vi "Database - Read.vi"(8 "error in (no error)":errorcluster, 11 "View Model":T1) -> (0 "error out":errorcluster, 3 "View Model":T1)   [LabVIEW 2017]
doc: "Reads the Configuration Database and store the information in an appropriate data structure.\n[Covers: SD3]"
uses:
  View Model/Controls/View Model.ctl
  View Model/Controls/Shared Model.ctl
  Error Handler/Controls/Error Model.ctl
  Error Handler/Controls/Error Message.ctl
  Error Handler/Controls/Error Level.ctl
  Controls/Database Model.ctl
  Controls/Database Message.ctl
  Controls/Database Command.ctl
  Controls/Database Overhead.ctl
  Controls/Database Status.ctl
  Controls/Database Record.ctl
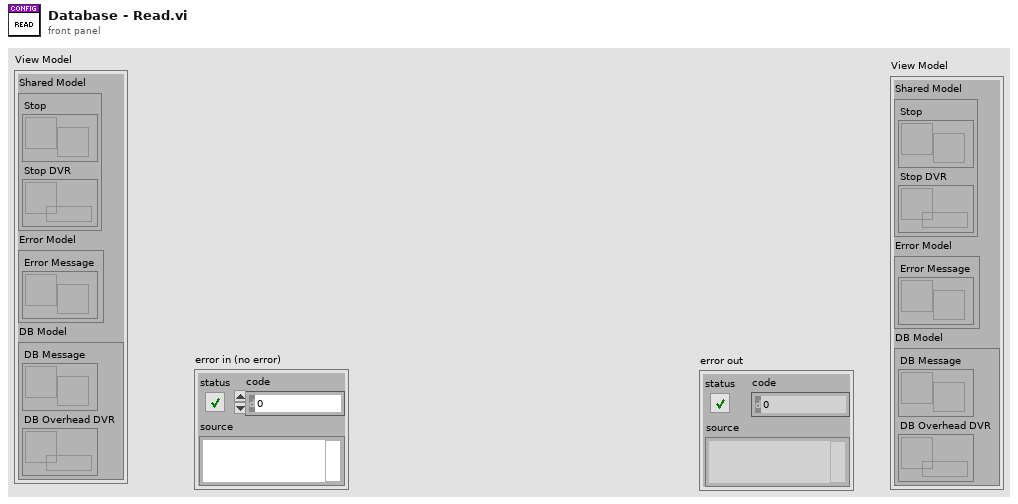
[diagram p1: front panel]
types:
  T1 = typedef "View Model.ctl" = cluster{"Shared Model":T2, "Error Model":T3, "DB Model":T4}
  T2 = typedef "Shared Model.ctl" = cluster{"Stop":refnum<user-event>, "Stop DVR":refnum<data-value>}
  T3 = typedef "Error Model.ctl" = cluster{"Error Message":refnum<user-event>}
  T4 = typedef "Database Model.ctl" = cluster{"DB Message":refnum<user-event>, "DB Overhead DVR":refnum<data-value>}
  T5 = typedef "Database Status.ctl" = enum16{"Unlocked", "Locked"}
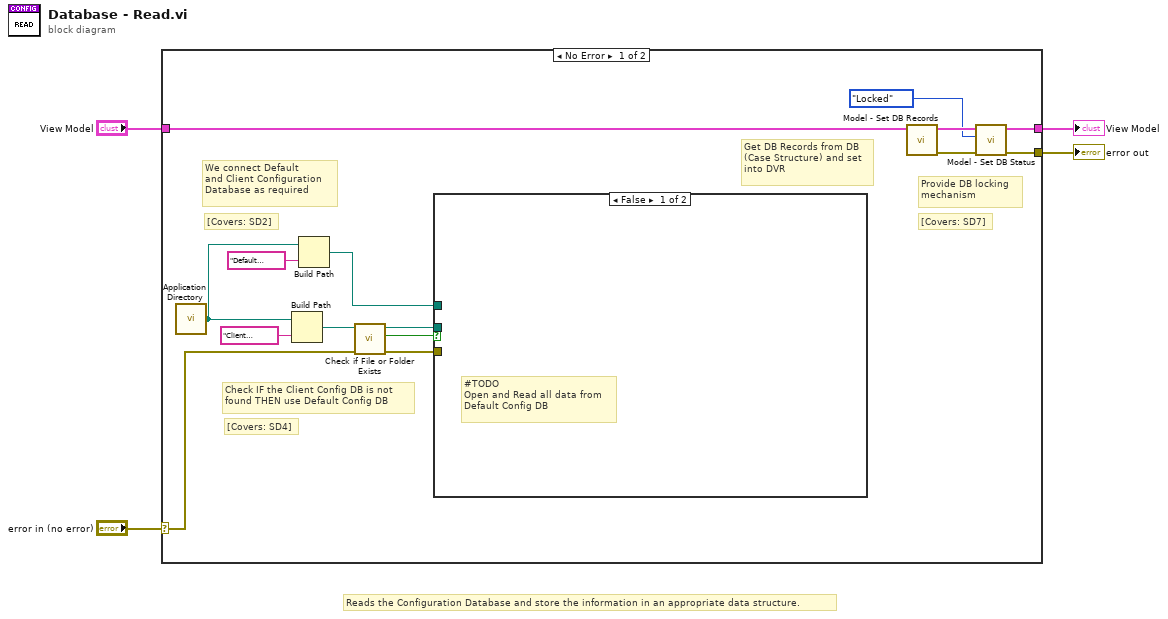
[diagram p0: block diagram]
diagram:
  # "Reads the Configuration Database and store the information in an appropriate data structure."
  n1 = case shown="No Error" "error in (no error)" {
    selector: "error in (no error)" -> [w12 w21]
    tunnel: "View Model" -> [w10 w20]
    tunnel: [w6 w20] -> w2
    tunnel: [w5 w21] -> w1
    frame No Error {
      # "Get DB Records from DB\n(Case Structure) and set\ninto DVR"
      # "[Covers: SD7]"
      # "Provide DB locking\nmechanism"
      # "[Covers: SD4]"
      # "Check IF the Client Config DB is not\nfound THEN use Default Config DB"
      # "[Covers: SD2]"
      # "We connect Default\nand Client Configuration\nDatabase as required"
      n2 = call <vilib>:"Application Directory.vi"() -> ("Application Directory"=w17:path)
      n3 = Build Path(base path=w17, name or relative path="Client Configuration Database.xml") -> (appended path=w16:path)
      n4 = Build Path(base path=w17, name or relative path="Default Configuration Database.xml") -> (appended path=w11:path)
      n5 = call <vilib>:"Check if File or Folder Exists.vi"("error in (no error)"=w12, "path"=w16) -> ("error out"=w13:errorcluster, "file or folder exists?"=w15:bool, "dup path"=w14:path)  [unwired: 7 in]
      n6 = case shown="False" w15 {
        tunnel: w14 -> [_ _]
        tunnel: w13 -> [_ _]
        tunnel: w11 -> [_ _]
        frame False {
          # "#TODO\nOpen and Read all data from\nDefault Config DB"
        }
        frame True {
          # "#TODO\nOpen and Read all data from\nClient Config DB"
        }
      }
      n7 = call "Model - Set DB Records.vi"("View Model"=w10) -> ("error out"=w8:errorcluster, "View Model"=w9:T1)  [unwired: 9 in]
      n8 = call "Model - Set DB Status.vi"("error in (no error)"=w8, "DB Status"=Database_Status."Locked", "View Model"=w9) -> ("error out"=w5:errorcluster, "View Model"=w6:T1)  [unwired: 7 in]
    }
    frame Error {
    }
  }
  "error out" <- w1
  "View Model" <- w2
